vi "setFPGAReference.vi"(10 "FPGAReference":refnum<k20>, 11 "MyHealthAndStatusWriteFIFO in":refnum<class "ModbusPort2WriteFIFO.lvclass">) -> (3 "MyHealthAndStatusWriteFIFO out":refnum<class "ModbusPort2WriteFIFO.lvclass">)   [LabVIEW 2015, in "ModbusPort2WriteFIFO.lvclass"]
uses:
  ModbusPort2WriteFIFO.lvclass
  ModbusPort2WriteFIFO.lvclass/ModbusPort2WriteFIFO.ctl
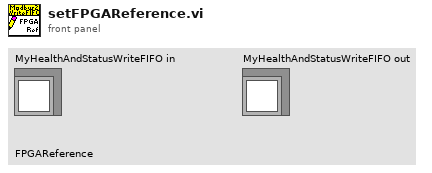
[diagram p1: front panel]
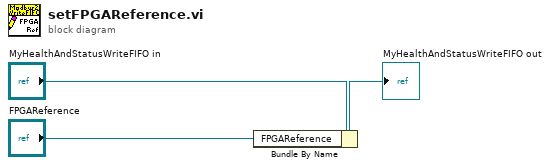
[diagram p0: block diagram]
diagram:
  n1 = Bundle By Name(cluster="MyHealthAndStatusWriteFIFO in", "FPGAReference"="FPGAReference") -> (→"MyHealthAndStatusWriteFIFO out":refnum<class "ModbusPort2WriteFIFO.lvclass">)
